vi "ZCAN_ReceiveLIN.vi"(4 "error in (no error)":errorcluster caption="错误输入（无错误）", 5 "ZCAN_LIN_MSG_WRAP":T1, 7 "channel_handle":u32) -> (0 "LIN数据帧数组":T1[](array[typedef]), 3 "Receive_Num":u32)   [LabVIEW 2020, in "zlgcan.lvlib"]
doc: "该函数用于接收CAN报文。"
uses:
  zlgcan.lvlib
  ZCAN_LIN_MSG.ctl
  bin/zlgcan_wrap.dll
  bin/zlgcan_wrap_LIN.dll
panel:
  out "缓冲区帧数":u32
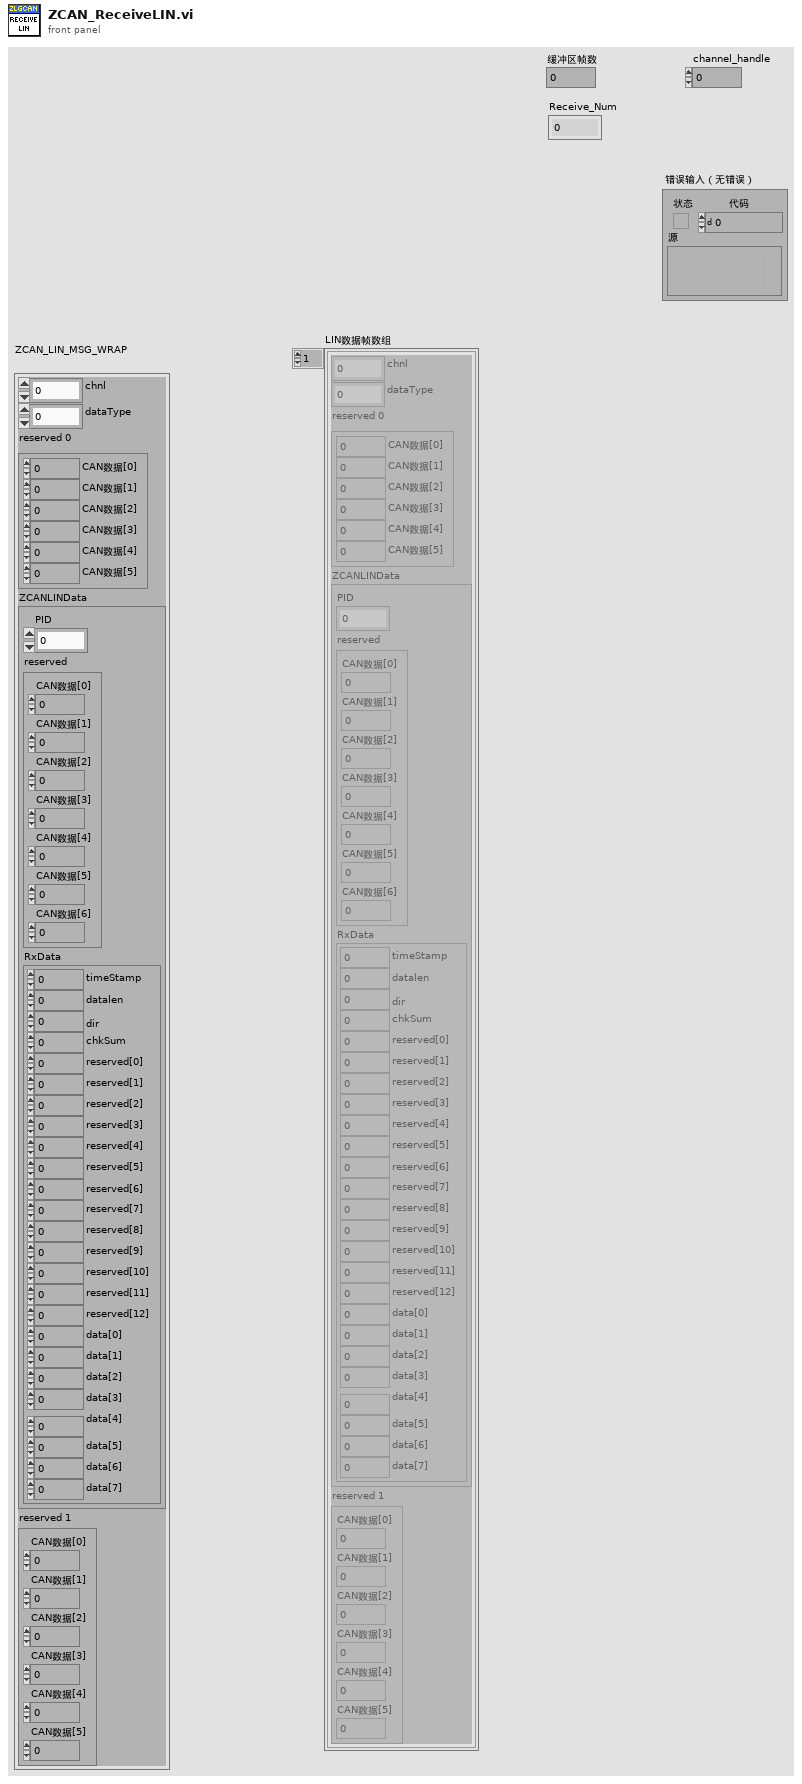
[diagram p1: front panel]
types:
  T1 = typedef "zlgcan.lvlib/ZCAN_LIN_MSG.ctl" = cluster{"chnl":u8, "dataType":u8, "reserved 0":cluster{"CAN数据[0]":u8, "CAN数据[1]":u8, "CAN数据[2]":u8, "CAN数据[3]":u8, "CAN数据[4]":u8, "CAN数据[5]":u8}, "ZCANLINData":cluster{"PID":u8, "reserved":cluster{"CAN数据[0]":u8, "CAN数据[1]":u8, "CAN数据[2]":u8, "CAN数据[3]":u8, "CAN数据[4]":u8, "CAN数据[5]":u8, "CAN数据[6]":u8}, "RxData":cluster{"timeStamp":u64, "datalen":u8, "dir":u8, "chkSum":u8, "reserved[0]":u8, "reserved[1]":u8, "reserved[2] ":u8, "reserved[3]":u8, "reserved[4]":u8, "reserved[5]":u8, "reserved[6] ":u8, "reserved[7] ":u8, "reserved[8]":u8, "reserved[9] ":u8, "reserved[10] ":u8, "reserved[11] ":u8, "reserved[12] ":u8, "data[0]":u8, "data[1]":u8, "data[2]":u8, "data[3]":u8, "data[4]":u8, "data[5]":u8, "data[6]":u8, "data[7]":u8}}, "reserved 1":cluster{"CAN数据[0]":u8, "CAN数据[1]":u8, "CAN数据[2]":u8, "CAN数据[3]":u8, "CAN数据[4]":u8, "CAN数据[5]":u8}}
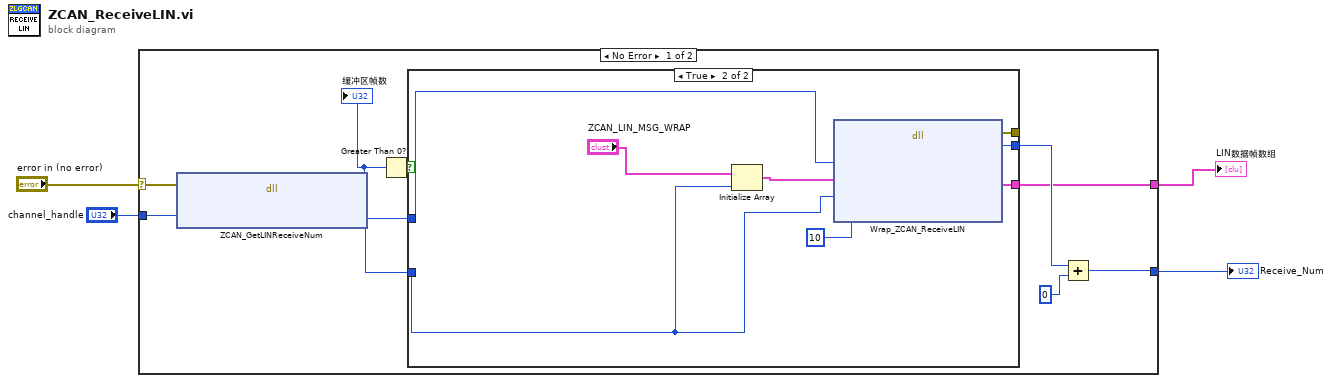
[diagram p0: block diagram]
diagram:
  n1 = case shown="No Error" "error in (no error)" {
    selector: "error in (no error)" -> [w13 _]
    tunnel: "channel_handle" -> [w9 _]
    tunnel: [w7 _] -> w2
    tunnel: [w6 _] -> w1
    frame No Error {
      n2 = dll-call lib="D:/Git/ZLG_USBCANFD/bin/zlgcan_wrap.dll" fn="ZCAN_GetLINReceiveNum"(error in=w13, "通道句柄"=w9) -> ("缓冲区帧数"=w10:u32, "通道句柄"=w11:u32)  [unwired: 2 in, 2 out]
      "缓冲区帧数" <- w10
      n3 = Greater Than 0?(x=w10) -> (x > 0?=w12:bool)
      n4 = case shown="True" w12 {
        tunnel: w11 -> [_ w20]
        tunnel: w10 -> [_ w14]
        tunnel: [_ w19] -> w6
        tunnel: [_ w18] -> _
        tunnel: [_ w17] -> w8
        frame False {
        }
        frame True {
          n5 = Initialize Array("ZCAN_LIN_MSG_WRAP", w14) -> (w16:T1[])
          n6 = dll-call lib="D:/Git/ZLG_USBCANFD/bin/zlgcan_wrap_LIN.dll" fn="Wrap_ZCAN_ReceiveLIN"("通道句柄"=w20, "数据帧数组"=w16, "数据帧数"=w14, "超时时间"=10) -> (error out=w18:errorcluster, "已接收帧数"=w17:u32, "数据帧数组"=w19:T1[])  [unwired: 6 in, 1 out]
        }
      }
      n7 = Add(x=w8, y=u32 0) -> (x+y=w7:u32)
    }
    frame Error {
    }
  }
  "Receive_Num" <- w2
  "LIN数据帧数组" <- w1
